vi "GetField.vi"(8 "error in (no error)":errorcluster, 9 "Instrument Ref In":refnum<k24>) -> (0 "Field\nStatus":i32(ring) items=["MagnetUnknown"=0, "StablePersistent"=1, "WarmingSwitch"=2, "CoolingSwitch"=3, "StableDriven"=4, "Iterating"=5, "Charging"=6, "Discharging"=7, "CurrentError"=8, "MagnetFailure"=15], 1 "Field":dbl, 2 "error out":errorcluster, 3 "Instrument Ref Out":refnum<k24>, 4 "GetField Error":i32)   [LabVIEW 2016]
uses:
  C:/user/patrick/git/PPMS-Monitor-and-Control/lvsrc/QDInstrument_LabView/QDInstrument.dll
  QDInstrument.dll
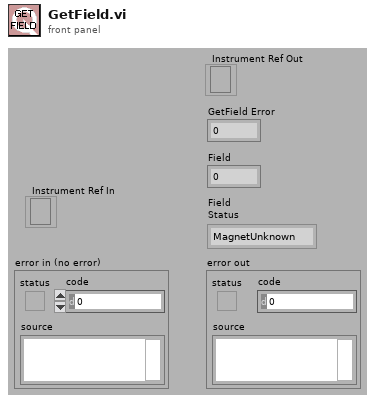
[diagram p1: front panel]
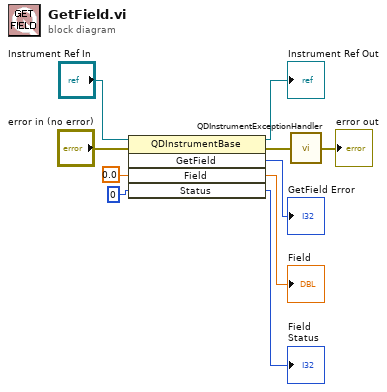
[diagram p0: block diagram]
diagram:
  n1 = invoke class="QDInstrumentBase" method="GetField"(reference="Instrument Ref In", error in="error in (no error)", "Field"=0.0 ("Temperature"), "Status"=0) -> (reference out=→"Instrument Ref Out":refnum<k24>, error out=w2:errorcluster, "GetField"=→"GetField Error":i32, "Field"=→"Field":dbl, "Status"=→"Field\nStatus":i32)  [unwired: 1 in]
  n2 = call "QDInstrumentExceptionHandler.vi"("Error in"=w2) -> ("Error out"=→"error out":errorcluster)
